vi "CameraRefNum_Simulation_Global.vi"(0 "menu":enum16{"set", "get", "delete"}(ring)=enum."get", 9 "Axis M1011 Set":refnum<k20>, 11 "error in (no error)":errorcluster) -> (10 "Axis M1011 Get":refnum<k20>, 15 "error out":errorcluster)   [LabVIEW 2017]
doc: "Sets a reference into a registry, gets a reference from a registry, or deletes a reference from a registry. The reference is accessed by name, and can be given any unique name.\n\nThis software is licensed. Open the labview\\readme\\WPI Robotics Library Open Source License.txt file for more information."
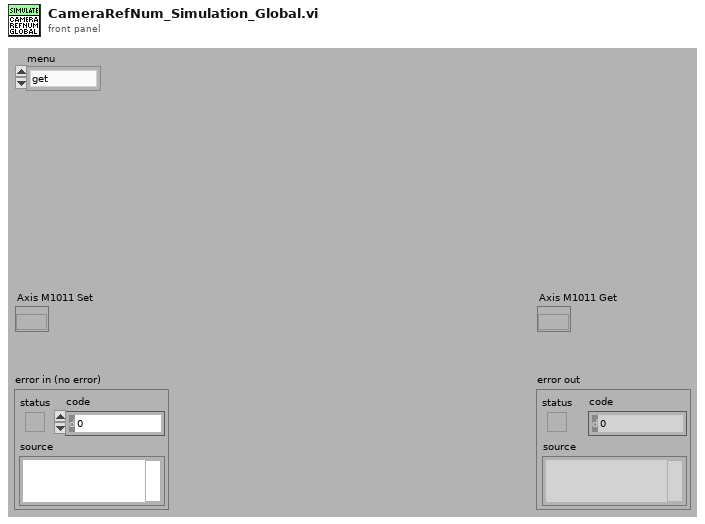
[diagram p1: front panel]
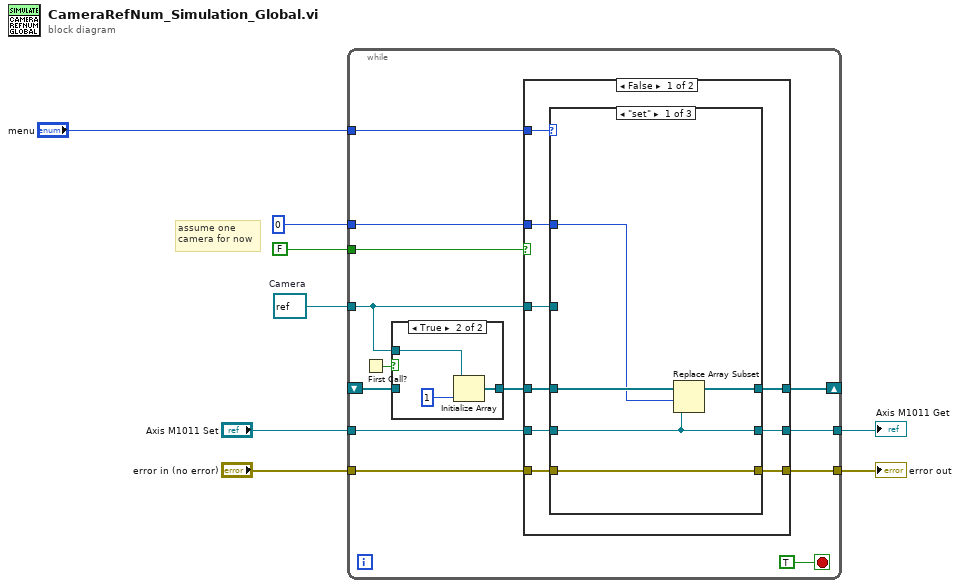
[diagram p0: block diagram]
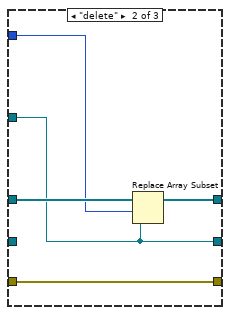
[diagram p2: hidden frame]
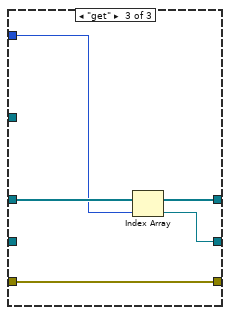
[diagram p3: hidden frame]
diagram:
  w5 = refnum<k20> refnum  # Camera
  # "assume one camera for now"
  n1 = while {
    tunnel: "Axis M1011 Set" -> [w21]
    tunnel: "error in (no error)" -> [w17]
    shift-right: [w20] -> _
    shift-left: _ -> [w12]
    tunnel: [w19] -> w3
    tunnel: "menu" -> [w18]
    tunnel: [w16] -> w7
    tunnel: u16 0 -> [w11]
    tunnel: FALSE ("result") -> [w10]
    tunnel: w5 -> [w9]
    stop <- TRUE stop-if-true
    n2 = First Call?() -> (First Call?: T/F=w14:bool)
    n3 = case shown="True" w14 {
      tunnel: [w48 w50] -> w13
      tunnel: w12 -> [w48 _]
      tunnel: w9 -> [_ w49]
      frame False {
      }
      frame True {
        n4 = Initialize Array(w49, 1 ("dimension size")) -> (w50:refnum<k20>[])
      }
    }
    n5 = case shown="False" w10 {
      tunnel: w21 -> [w30 _]
      tunnel: [w29 w47] -> w20
      tunnel: [w28 w45] -> w19
      tunnel: w18 -> [w27 _]
      tunnel: w17 -> [w26 w46]
      tunnel: [w25 w46] -> w16
      tunnel: w13 -> [w24 w47]
      tunnel: w11 -> [w23 _]
      tunnel: w9 -> [w22 w45]
      frame False {
        n6 = case shown="\"set\"" w27 {
          tunnel: w30 -> [w33 _ _]
          tunnel: [w34 w39 w44] -> w29
          tunnel: w24 -> [w35 w40 w44]
          tunnel: [w33 w36 w43] -> w28
          tunnel: [w32 w38 w42] -> w25
          tunnel: w26 -> [w32 w38 w42]
          tunnel: w23 -> [w31 w37 w41]
          tunnel: w22 -> [_ w36 _]
          frame "set" {
            n7 = Replace Array Subset(array=w35, new element=w33, index=w31) -> (w34:refnum<k20>[])
          }
          frame "delete" {
            n8 = Replace Array Subset(array=w40, new element=w36, index=w37) -> (w39:refnum<k20>[])
          }
          frame "get" {
            n9 = Index Array(array=w44, index=w41) -> (element=w43:refnum<k20>)
          }
        }
      }
      frame True {
        # "Do nothing if different modules."
        # "Do nothing if channel is Invalid."
      }
    }
  }
  "error out" <- w7
  "Axis M1011 Get" <- w3
